vi "CreateTable.vi"(7 "Drop?":bool, 8 "error in (no error)":errorcluster, 9 "Items":string[](array[string]), 10 "Table Name":string, 11 "SQLite Connection in":refnum<class "Connection.lvclass">) -> (0 "error out":errorcluster, 3 "SQLite Connection out":refnum<class "Connection.lvclass">)   [LabVIEW 2015, in "DBToolkit.lvlib"]
uses:
  DBToolkit.lvlib
  <vilib>/drjdpowell/SQLite Library/SQL Connection/Connection.lvclass
  <vilib>/drjdpowell/SQLite Library/SQL Connection/Execute SQL (No results).vi
  <vilib>/drjdpowell/SQLite Library/SQLite.lvlib
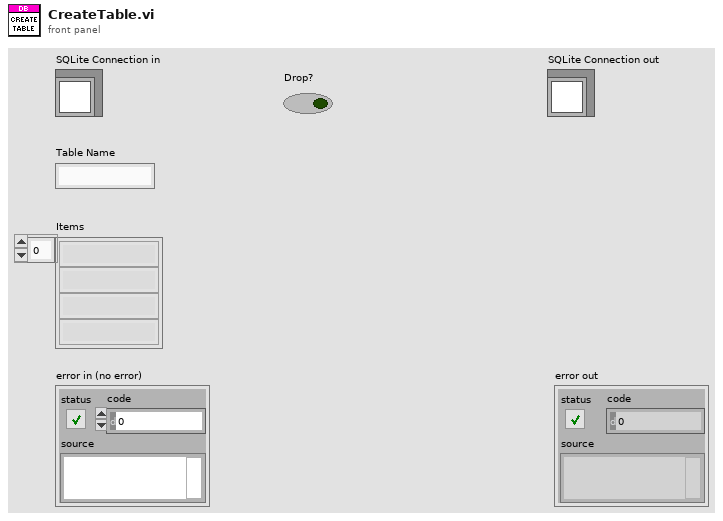
[diagram p1: front panel]
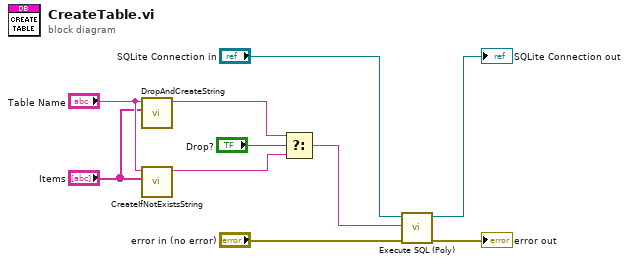
[diagram p0: block diagram]
diagram:
  n1 = call "DropAndCreateString.vi"("Items"="Items", "Table Name"="Table Name") -> ("Drop and Create String"=w9:string)  [unwired: 9 in]
  n2 = call "CreateIfNotExistsString.vi"("Items"="Items", "Table Name"="Table Name") -> ("Create If Not Existed String"=w8:string)  [unwired: 9 in]
  n3 = Select(t=w9, s="Drop?", f=w8) -> (s? t:f=w6:string)
  n4 = call-poly <vilib>:"Execute SQL (Poly).vi"("error in (no error)"="error in (no error)", "SQL"=w6, "SQLite Connection in"="SQLite Connection in") -> ("error out"=→"error out":errorcluster, "SQLite Connection out"=→"SQLite Connection out":refnum<class "Connection.lvclass">)  [unwired: 7 in]
